vi "TLB Native Dynamic Events ver 0.04e.vi"() -> ()   [LabVIEW 2018]
uses:
  Labview Training Phase 2/Enum Controls/States for Action Engine.ctl
  Type def/TLB event states.ctl
  Type def/TLB MHL States.ctl
  <vilib>/Studica/Studica Toolkit/Background/I2C Channel.ctl
  <vilib>/Studica/Studica Toolkit/NavX/NavX.lvlib
  <vilib>/myRIO/Common/Instrument Driver Framework/myRIO v1.0/AI/typedefs/AI Channels Enum.ctl
  <vilib>/myRIO/Common/Instrument Driver Framework/myRIO v1.0/AI/typedefs/AI Channels List.ctl
  <vilib>/Studica/Studica Toolkit/Background/Mxp Selection.ctl
  <vilib>/ptbypt/NI_PtbyPt.lvlib
panel:
  out "NavX Info Out":T2
  out "LinearAcceleration":T3
  out "Displacement":T4
  out "YRPHfH":T5
  in  "y":dbl=-1.2 format="%#_13g"
  out "Distance":T6
  in  "Return to IDLE":bool
  out "Sharp IR Distance":dbl
  out "Sharp IR Distance 2":dbl
  out "CM":fxp<+,64,16>
  out "Ultrasonic sensor":dbl format="%0.2f"
  out "Waveform Chart 3":dbl(graph)
  in  "xTargetSpeed":dbl
  in  "yTargetSpeed":dbl
  in  "wTargetSpeed":dbl
  out "Speed":T7
  in  "Reset Encoder 0":bool
  out "Action Queue Items":i32
  out "State Logic Queue Items":i32
  out "Action Queues items":string[](array[string])=["Hardware reset", "Software reset", ""]
  out "State logic":T8=enum."Task 2"
  out "Action State":string
  in  "Tasks Selector":string(combo)="Task 2"
  in  "Stop Queue":bool
  in  "Start Task":bool
  # "Test Programme written by Calvin Loke    Dated: 28 Aug 2019\nTest Programme revised by Dr Alex See   Dated 30 Aug 2019\n\nProgramme version:   TLB Native Dynamic Events ver 0.04b.vi"
  # "System Health Status Update"
  # "Sequence of Actions"
  # "Continuous (Repeated)"
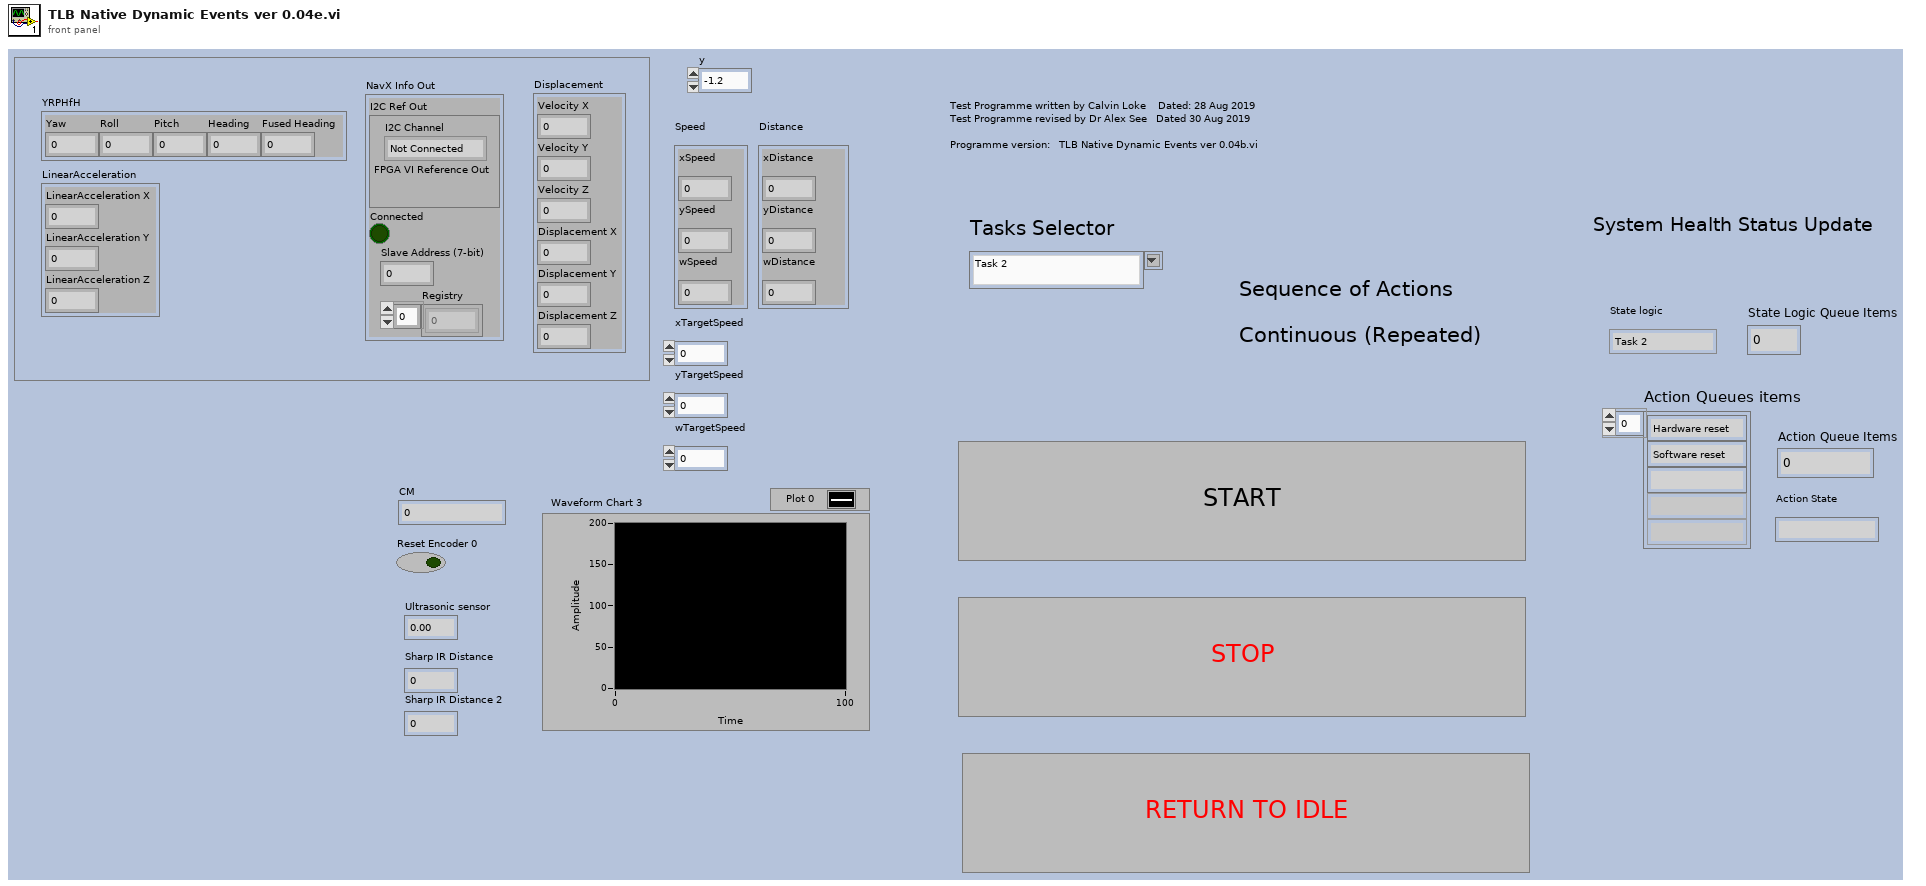
[diagram p1: front panel]
types:
  T1 = typedef "I2C Channel.ctl" = enum16{"Not Connected", "A", "B"}
  T2 = cluster{"I2C Ref Out":cluster{"I2C Channel":T1, "FPGA VI Reference Out":refnum<k20>}, "Connected":bool, "Slave Address (7-bit)":u8, "Registry":u8[]}
  T3 = cluster{"LinearAcceleration X":dbl, "LinearAcceleration Y":dbl, "LinearAcceleration Z":dbl}
  T4 = cluster{"Velocity X":dbl, "Velocity Y":dbl, "Velocity Z":dbl, "Displacement X":dbl, "Displacement Y":dbl, "Displacement Z":dbl}
  T5 = cluster{"Yaw":dbl, "Roll":dbl, "Pitch":dbl, "Heading":dbl, "Fused Heading":dbl}
  T6 = cluster{"xDistance":dbl, "yDistance":dbl, "wDistance":dbl}
  T7 = cluster{"xSpeed":dbl, "ySpeed":dbl, "wSpeed":dbl}
  T8 = typedef "TLB MHL States.ctl" = enum16{"None", "Startup", "Idle", "Processing", "Shutdown", "Reset", "Task 1", "Task 2", "Task 3", "Task 4", "Task 4a", "Task 4b", "Task 4c", "Task 4d", "Task 4e", "Task 4f", "Task 4g", "Task 4h", "Acquire image", "Wall follow mode", "Autodrive", "Autodrive a"}
  T9 = typedef "States for Action Engine.ctl" = enum16{"Initialize", "Write", "Read"}
  T10 = typedef "TLB event states.ctl" = enum16{"Start Sequence", "Exit", "Start Task 1", "Start Task 2", "Start Task 3", "Start Task 4", "Camera vision", "Wall follow mode", "Idle", "Start Drive Straight"}
  T11 = typedef "Mxp Selection.ctl" = enum16{"MXP A", "MXP B"}
  T12 = typedef "TLB event states.ctl" = enum16{"Start Sequence", "Exit", "Task 1", "Task 2", "Task 3", "Idle"}
  T13 = typedef "AI Channels List.ctl" = T14[]
  T14 = typedef "AI Channels Enum.ctl" = enum16{"Not Connected", "AudioIn/Left", "AudioIn/Right", "C/AI0", "C/AI1", "A/AI0", "A/AI1", "A/AI2", "A/AI3", "A/AI4", "A/AI5", "A/AI6", "A/AI7", "B/AI0", "B/AI1", "B/AI2", "B/AI3", "B/AI4", "B/AI5", "B/AI6", "B/AI7", "AI/AI0", "AI/AI1", "AI/AI2", "AI/AI3", "A/AI0 (DIFF)", "A/AI1 (DIFF)", "A/AI2 (DIFF)", "A/AI3 (DIFF)", "B/AI0 (DIFF)", "B/AI1 (DIFF)", "B/AI2 (DIFF)", "B/AI3 (DIFF)"}
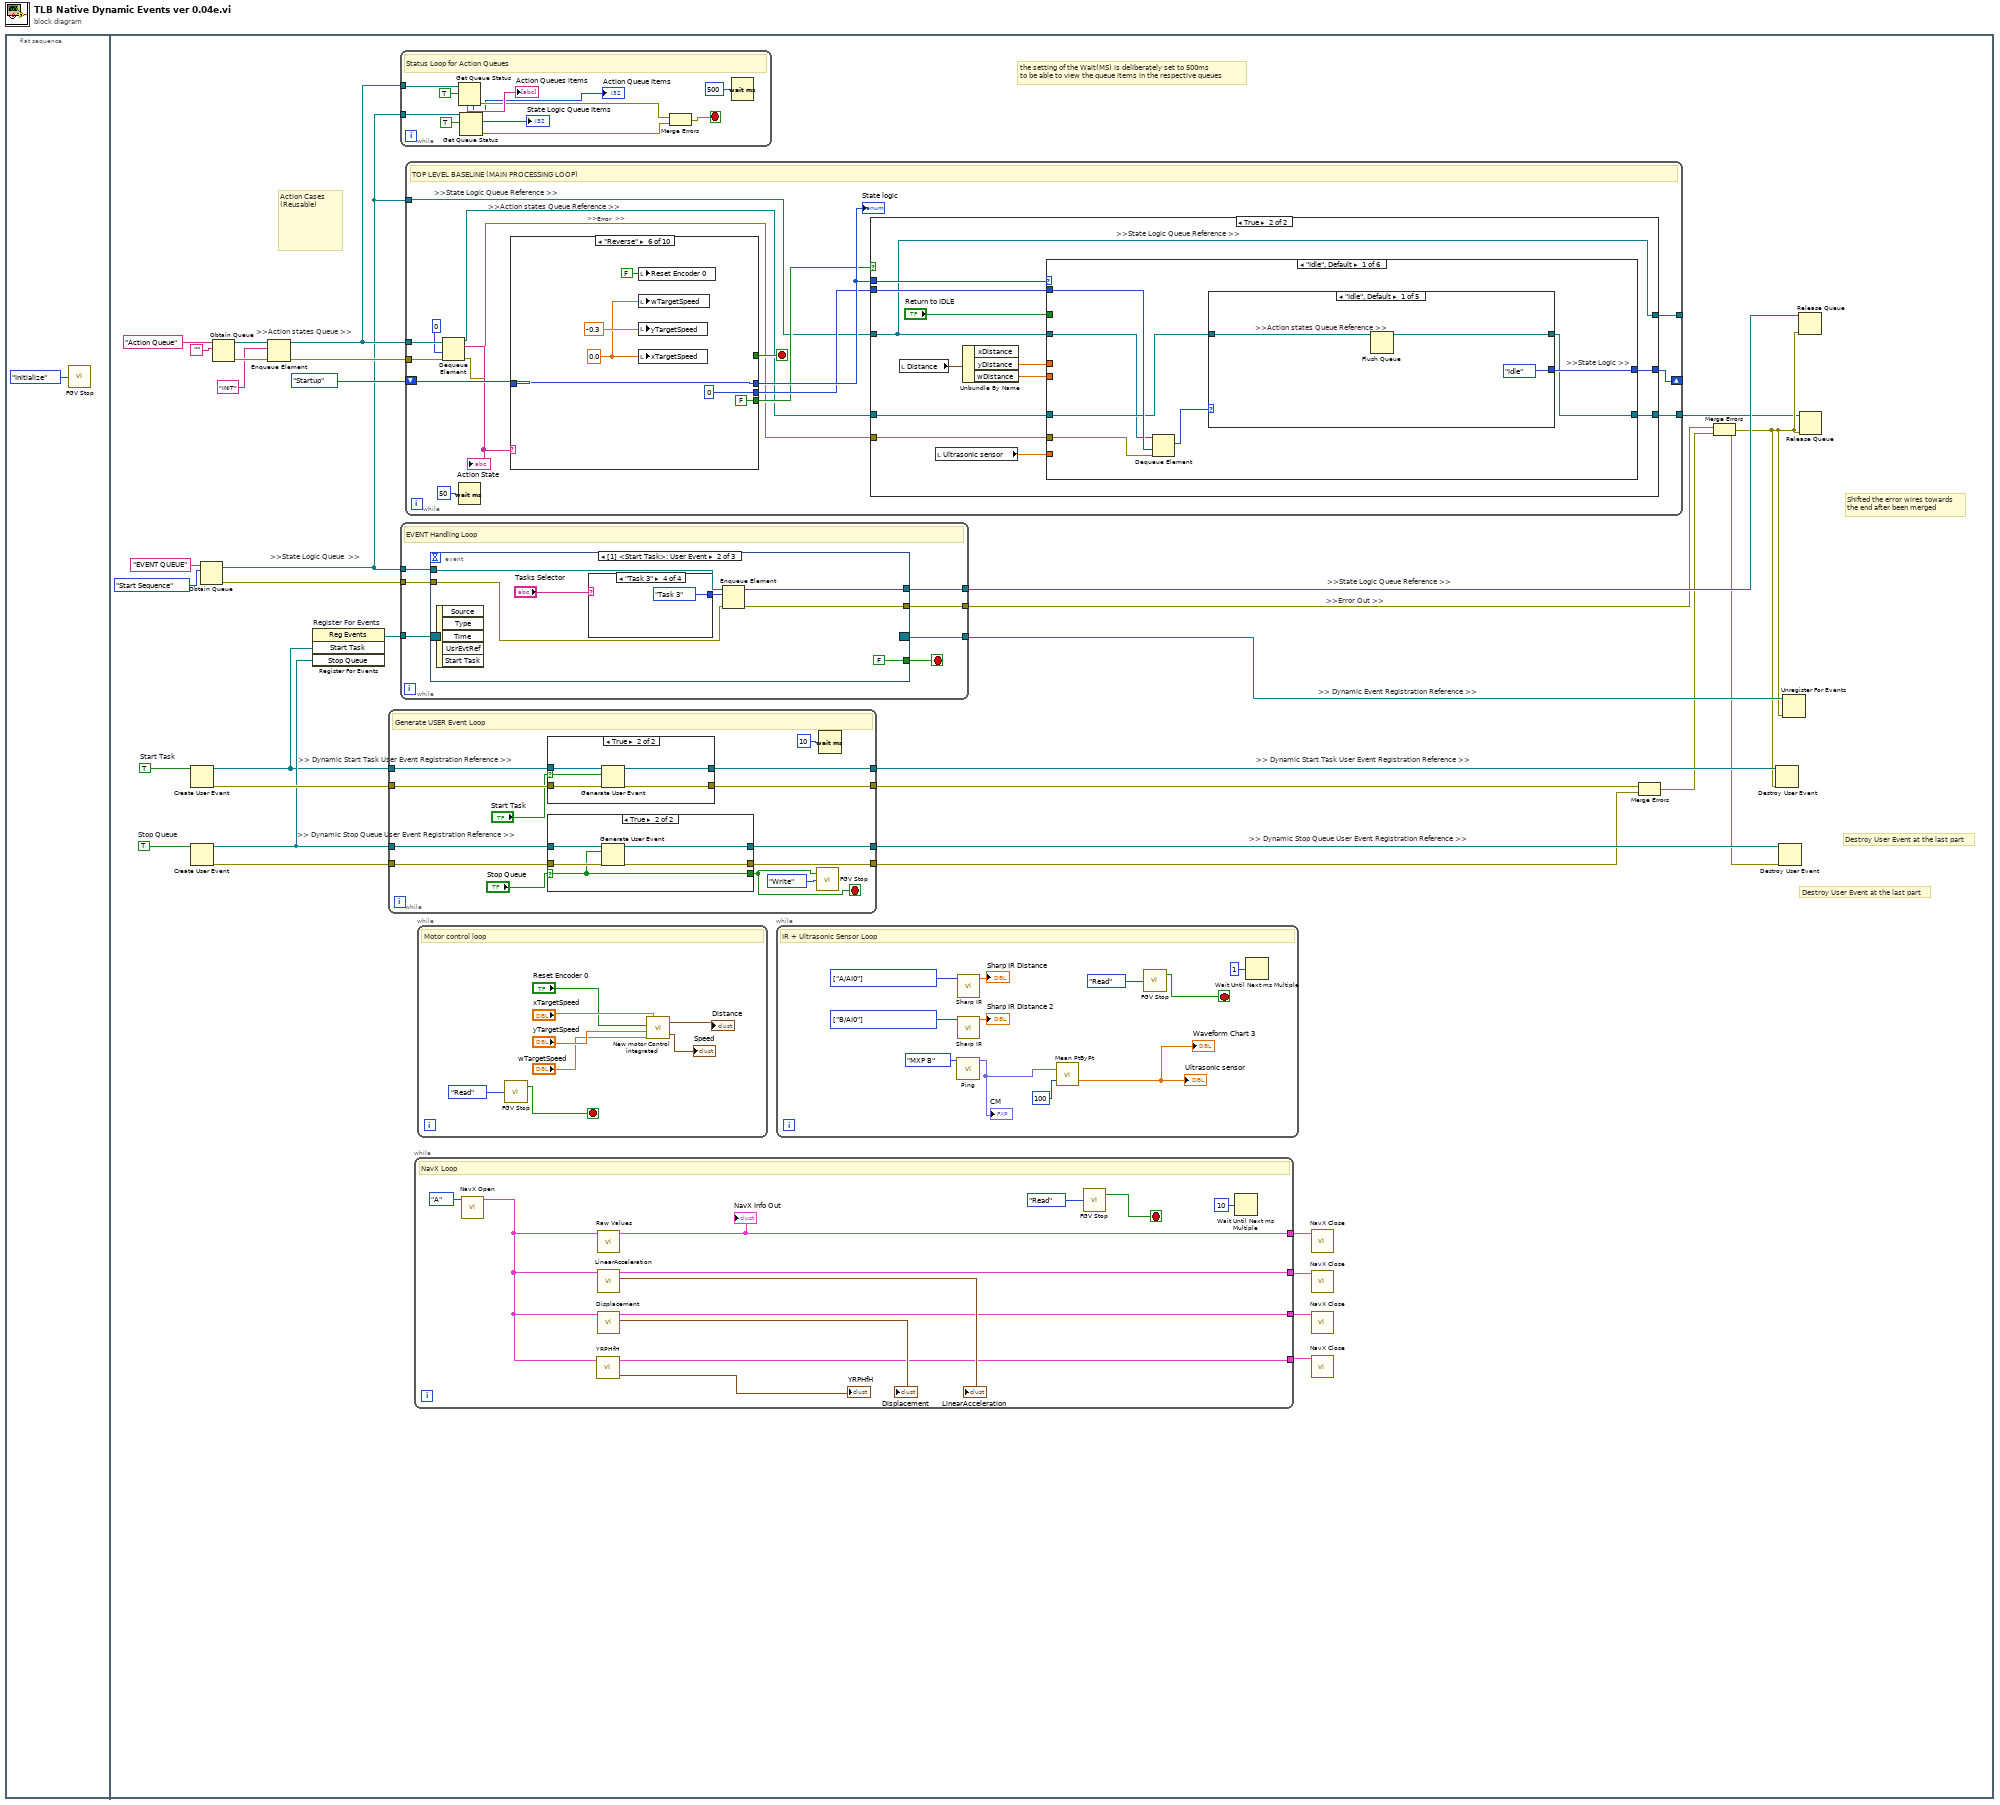
[diagram p0: block diagram]
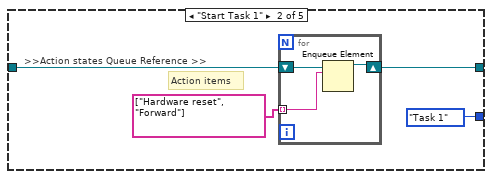
[diagram p3: hidden frame]
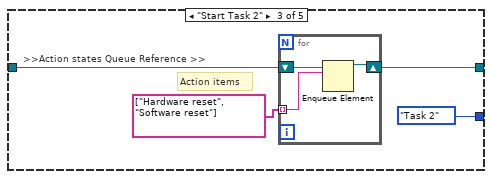
[diagram p4: hidden frame]
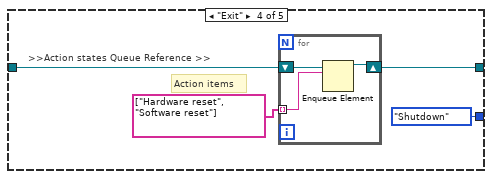
[diagram p5: hidden frame]
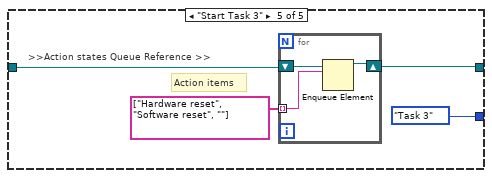
[diagram p6: hidden frame]
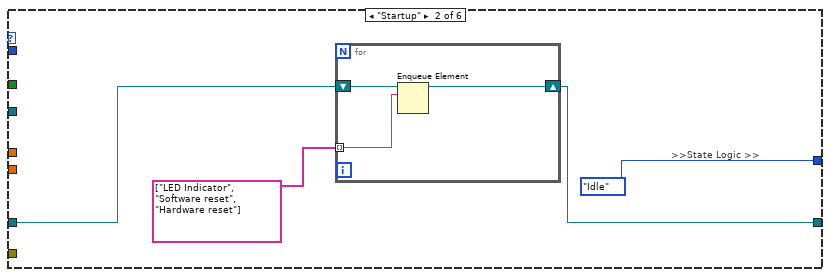
[diagram p7: hidden frame]
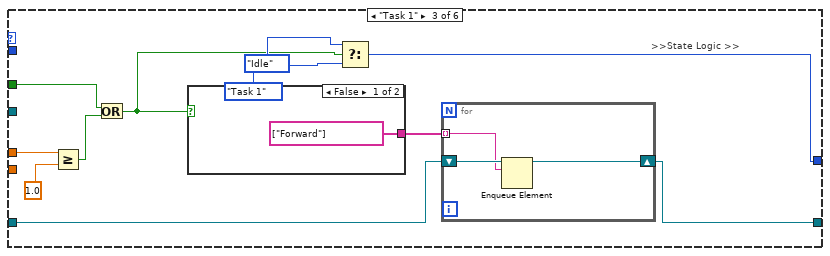
[diagram p8: hidden frame]
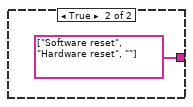
[diagram p9: hidden frame]
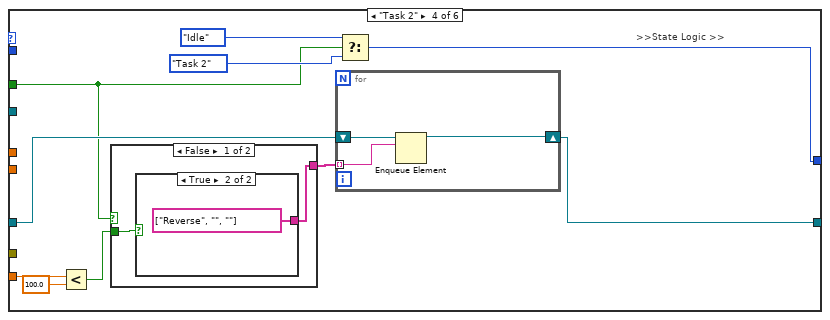
[diagram p10: hidden frame]
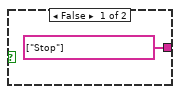
[diagram p11: hidden frame]
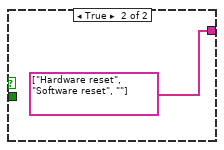
[diagram p12: hidden frame]
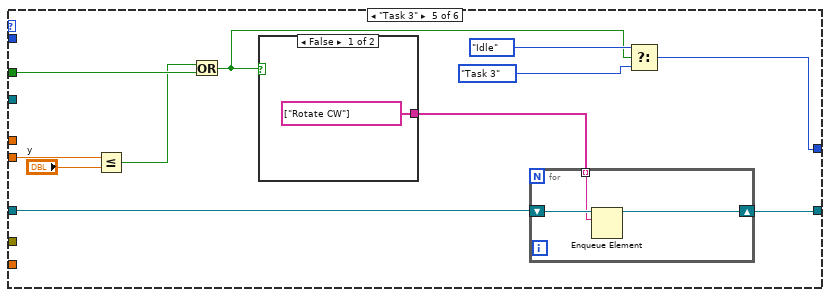
[diagram p13: hidden frame]
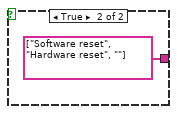
[diagram p14: hidden frame]
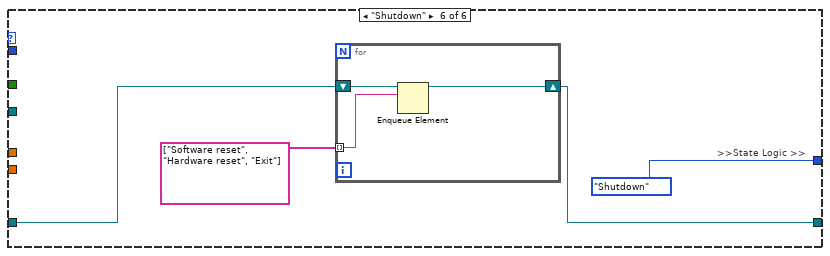
[diagram p15: hidden frame]
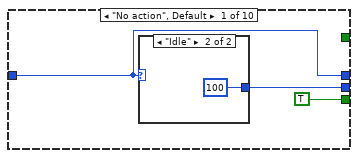
[diagram p16: hidden frame]
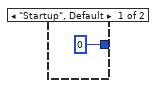
[diagram p17: hidden frame]
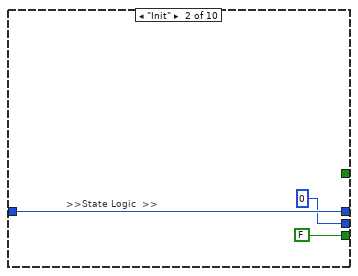
[diagram p18: hidden frame]
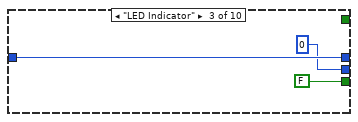
[diagram p19: hidden frame]
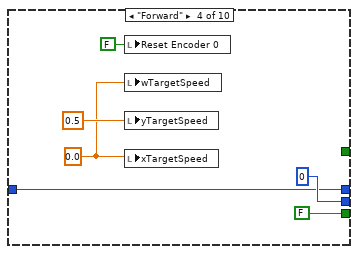
[diagram p20: hidden frame]
diagram:
  n1 = flat-sequence {
    frame #0 {
      n2 = call "FGV Stop.vi"("Init/Read/Write State"=States_for_Action_Engine."Initialize") -> ()  [unwired: 2 in, 2 out]
    }
    frame #1 {
      w34 = TRUE  # Stop Queue
      w33 = TRUE  # Start Task
      # "the setting of the Wait(MS) is deliberately set to 500ms\nto be able to view the queue items in the respective queues"
      # "Action Cases\n(Reusable)"
      # ">>Error Out >>"
      # ">> Dynamic Stop Queue User Event Registration Reference >>"
      # ">> Dynamic Start Task User Event Registration Reference >>"
      # ">> Dynamic Stop Queue User Event Registration Reference >>"
      # ">> Dynamic Start Task User Event Registration Reference >>"
      # ">> Dynamic Event Registration Reference >>"
      # ">>Action states Queue >>"
      # ">>State Logic Queue  >>"
      # ">>State Logic Queue Reference >>"
      # "Destroy User Event at the last part"
      # "Destroy User Event at the last part"
      # "Shifted the error wires towards\nthe end after been merged"
      n3 = Create User Event(user event datatype=w33) -> (user event=w25:refnum<user-event>, error out=w30:errorcluster)  [unwired: 1 in]
      n4 = Create User Event(user event datatype=w34) -> (user event=w26:refnum<user-event>, error out=w29:errorcluster)  [unwired: 1 in]
      n5 = Obtain Queue(name (unnamed)="EVENT QUEUE", element data type=TLB_event_states."Start Sequence" ("Enum")) -> (queue out=w9:refnum<queue>, error out=w15:errorcluster)  [unwired: 3 in, 1 out]
      n6 = Obtain Queue(name (unnamed)="Action Queue", element data type="") -> (queue out=w18:refnum<queue>, error out=w14:errorcluster)  [unwired: 3 in, 1 out]
      n7 = Enqueue Element(queue=w18, element="INIT", error in (no error)=w14) -> (queue out=w10:refnum<queue>, error out=w13:errorcluster)  [unwired: 1 in, 1 out]
      n8 = register-events "Register For Events"(w25, w26) -> (reference out=w24:refnum<event-registration>)  [unwired: 2 in, 1 out]
      n9 = while {
        tunnel: w25 -> [w297]
        tunnel: w26 -> [w296]
        tunnel: [w295] -> w32
        tunnel: [w294] -> w31
        tunnel: w30 -> [w293]
        tunnel: [w292] -> w28
        tunnel: w29 -> [w291]
        tunnel: [w290] -> w27
        stop <- w286 stop-if-true
        # "Generate USER Event Loop"
        n10 = case shown="True" "Start Task" {
          selector: "Start Task" -> [_ w309]
          tunnel: w297 -> [w308 w313]
          tunnel: [w308 w312] -> w294
          tunnel: w293 -> [w307 w311]
          tunnel: [w307 w310] -> w292
          frame False {
          }
          frame True {
            n11 = Generate User Event(user event=w313, event data cluster=w309, error in=w311) -> (user event out=w312:refnum<user-event>, error out=w310:errorcluster)  [unwired: 1 in]
          }
        }
        n12 = case shown="True" "Stop Queue" {
          selector: "Stop Queue" -> [_ w302]
          tunnel: w296 -> [w301 w306]
          tunnel: [w301 w305] -> w295
          tunnel: w291 -> [w300 w304]
          tunnel: [w300 w303] -> w290
          tunnel: [FALSE w302] -> w286
          frame False {
          }
          frame True {
            n13 = Generate User Event(user event=w306, event data cluster=w302, error in=w304) -> (user event out=w305:refnum<user-event>, error out=w303:errorcluster)  [unwired: 1 in]
          }
        }
        n14 = call "FGV Stop.vi"("Init/Read/Write State"=States_for_Action_Engine."Write", "Input Node"=w286) -> ()  [unwired: 1 in, 2 out]
        n15 = Wait (ms)(milliseconds to wait=u32 10) -> ()  [unwired: 1 out]
      }
      n16 = while {
        tunnel: w10 -> [w74]
        tunnel: w9 -> [w71]
        stop <- w68 stop-if-true
        # "Status Loop for Action Queues"
        n17 = Get Queue Status(queue=w74, return elements? (F)=TRUE) -> (error out=w70:errorcluster, # elements in queue=→"Action Queue Items":i32, elements=→"Action Queues items":string[])  [unwired: 1 in, 5 out]
        n18 = Get Queue Status(queue=w71, return elements? (F)=TRUE) -> (# pending remove=→"State Logic Queue Items":i32, error out=w69:errorcluster)  [unwired: 1 in, 6 out]
        n19 = Merge Errors(w70, w69) -> (w68:errorcluster)
        n20 = Wait (ms)(milliseconds to wait=u32 500) -> ()  [unwired: 1 out]
      }
      n21 = while {
        tunnel: w24 -> [w262]
        tunnel: [w261] -> w23
        tunnel: w9 -> [w259]
        tunnel: [w258] -> w22
        tunnel: w15 -> [w257]
        tunnel: [w256] -> w12
        stop <- w260 stop-if-true
        # "EVENT Handling Loop"
        n22 = event shown="[1] <Start Task>: User Event" {
          selector: w262 -> [_ _ _]
          dyn-events: [_ _ _] -> w261
          timeout: _ -> [_ _ _]
          tunnel: [FALSE FALSE w285] -> w260
          tunnel: w259 -> [w267 w274 w283]
          tunnel: [w266 w273 w284] -> w258
          tunnel: w257 -> [w264 w270 w281]
          tunnel: [w263 w269 w280] -> w256
          event Timeout {
            n23 = event-data() -> ()  [unwired: 1 in, 3 out]
            n24 = Enqueue Element(queue=w267, element=TLB_event_states."Idle" ("Enum"), error in (no error)=w264) -> (queue out=w266:refnum<queue>, error out=w263:errorcluster)  [unwired: 1 in, 1 out]
          }
          event User Event {
            n25 = event-data() -> ()  [unwired: 1 in, 5 out]
            n26 = case shown="\"Task 3\"" "Tasks Selector" {
              tunnel: [TLB_event_states."Idle" ("Enum") TLB_event_states."Start Task 1" ("Enum") TLB_event_states."Task 2" ("Enum") TLB_event_states."Task 3" ("Enum")] -> w271
              frame Default {
              }
              frame "Task 1" {
              }
              frame "Task 2" {
              }
              frame "Task 3" {
              }
            }
            n27 = Enqueue Element(queue=w274, element=w271, error in (no error)=w270) -> (queue out=w273:refnum<queue>, error out=w269:errorcluster)  [unwired: 1 in, 1 out]
          }
          event User Event {
            n28 = event-data() -> ("Stop Queue"=w285:bool)  [unwired: 1 in, 4 out]
            n29 = Enqueue Element At Opposite End(queue=w283, element=TLB_event_states."Exit" ("Enum"), error in (no error)=w281) -> (queue out=w284:refnum<queue>, error out=w280:errorcluster)  [unwired: 1 in, 1 out]
          }
        }
      }
      n30 = while {
        tunnel: w9 -> [w79]
        shift-right: [w84] -> _
        shift-left: TLB_MHL_States."Startup" ("Enum") -> [w91]
        tunnel: w10 -> [w89]
        tunnel: w13 -> [w87]
        tunnel: [w86] -> _
        tunnel: [w85] -> w7
        stop <- w82 stop-if-true
        # ">>Error  >>"
        # ">>Action states Queue Reference >>"
        # ">>State Logic Queue Reference >>"
        # "TOP LEVEL BASELINE (MAIN PROCESSING LOOP)"
        n31 = Dequeue Element(queue=w89, timeout in ms (-1)=0, error in (no error)=w87) -> (queue out=w78:refnum<queue>, element=w88:string, error out=w77:errorcluster)  [unwired: 1 out]
        "Action State" <- w88
        n32 = Wait (ms)(milliseconds to wait=u32 50) -> ()  [unwired: 1 out]
        n33 = case shown="\"Reverse\"" w88 {
          tunnel: [w212 w217 w220 w225 w230 w237 w242 w246 w251 TLB_MHL_States."Shutdown" ("Enum")] -> w90
          tunnel: w91 -> [w212 w217 w220 w225 w230 w237 w242 w246 w251 _]
          tunnel: [w211 0 0 0 0 0 0 0 0 0] -> w83
          tunnel: [_ _ _ _ _ _ _ _ _ TRUE] -> w82
          tunnel: [TRUE FALSE FALSE FALSE FALSE FALSE FALSE FALSE FALSE FALSE] -> w81
          frame "No action", Default {
            n34 = case shown="\"Idle\"" w212 {
              tunnel: [0 100] -> w211
              frame "Startup", Default {
              }
              frame "Idle" {
              }
            }
          }
          frame "Init" {
            # ">>State Logic  >>"
          }
          frame "LED Indicator" {
          }
          frame "Forward" {
            w221 = 0.0
            n35 = local write "Reset Encoder 0"(FALSE ("Reset Encoder 0")) -> ()
            n36 = local write "wTargetSpeed"(w221) -> ()
            n37 = local write "yTargetSpeed"(0.5 ("yTargetSpeed")) -> ()
            n38 = local write "xTargetSpeed"(w221) -> ()
          }
          frame "Rotate CW" {
            w227 = 0.0
            n39 = local write "Reset Encoder 0"(FALSE ("Reset Encoder 0")) -> ()
            n40 = local write "wTargetSpeed"(-0.15 ("yTargetSpeed")) -> ()
            n41 = local write "yTargetSpeed"(w227) -> ()
            n42 = local write "xTargetSpeed"(w227) -> ()
          }
          frame "Reverse" {
            w233 = 0.0
            n43 = local write "Reset Encoder 0"(FALSE ("Reset Encoder 0")) -> ()
            n44 = local write "wTargetSpeed"(w233) -> ()
            n45 = local write "yTargetSpeed"(-0.3 ("yTargetSpeed")) -> ()
            n46 = local write "xTargetSpeed"(w233) -> ()
          }
          frame "Stop" {
            w239 = 0.0
            n47 = local write "Reset Encoder 0"(FALSE ("Reset Encoder 0")) -> ()
            n48 = local write "wTargetSpeed"(w239) -> ()
            n49 = local write "yTargetSpeed"(w239) -> ()
            n50 = local write "xTargetSpeed"(w239) -> ()
          }
          frame "Software reset" {
          }
          frame "Hardware reset" {
            w247 = 0.0
            n51 = local write "Reset Encoder 0"(TRUE ("Reset Encoder 0")) -> ()
            n52 = local write "wTargetSpeed"(w247) -> ()
            n53 = local write "yTargetSpeed"(w247) -> ()
            n54 = local write "xTargetSpeed"(w247) -> ()
          }
          frame "Exit" {
          }
        }
        "State logic" <- w90
        n55 = case shown="True" w81 {
          tunnel: w90 -> [w94 w107]
          tunnel: w79 -> [w95 w101]
          tunnel: w78 -> [w93 w106]
          tunnel: [w95 w101] -> w86
          tunnel: [w93 w105] -> w85
          tunnel: [w94 w104] -> w84
          tunnel: w77 -> [_ w103]
          tunnel: w83 -> [_ w102]
          frame False {
          }
          frame True {
            # ">>State Logic Queue Reference >>"
            n56 = local read "Distance"() -> (w99:T6)
            n57 = local read "Ultrasonic sensor"() -> (w97:dbl)
            n58 = Unbundle By Name(w99) -> ("yDistance"=w98:dbl, "wDistance"=w96:dbl)  [unwired: 1 out]
            n59 = case shown="\"Idle\", Default" w107 {
              tunnel: w101 -> [w108 _ _ _ _ _]
              tunnel: w106 -> [w110 w147 w159 w174 w196 w204]
              tunnel: [w109 w146 w158 w175 w195 w203] -> w105
              tunnel: [w113 TLB_MHL_States."Idle" ("Enum") w161 w176 w192 TLB_MHL_States."Shutdown" ("Enum")] -> w104
              tunnel: w103 -> [w111 _ _ _ _ _]
              tunnel: w102 -> [w112 _ _ _ _ _]
              tunnel: "Return to IDLE" -> [_ _ w156 w171 w190 _]
              tunnel: w98 -> [_ _ w155 _ _ _]
              tunnel: w97 -> [_ _ _ w173 _ _]
              tunnel: w96 -> [_ _ _ _ w189 _]
              frame "Idle", Default {
                # ">>State Logic >>"
                n60 = Dequeue Element(queue=w108, timeout in ms (-1)=w112, error in (no error)=w111) -> (element=w114:T10)  [unwired: 3 out]
                n61 = case shown="\"Idle\", Default" w114 {
                  tunnel: [TLB_MHL_States."Idle" ("Enum") TLB_MHL_States."Task 1" ("Enum") TLB_MHL_States."Task 2" ("Enum") TLB_MHL_States."Shutdown" ("Enum") TLB_MHL_States."Task 3" ("Enum")] -> w113
                  tunnel: [w115 w120 w125 w132 w141] -> w109
                  tunnel: w110 -> [w116 w118 w126 w133 w142]
                  frame "Idle", Default {
                    # ">>Action states Queue Reference >>"
                    n62 = Flush Queue(queue=w116) -> (queue out=w115:refnum<queue>)  [unwired: 1 in, 2 out]
                  }
                  frame "Start Task 1" {
                    # ">>Action states Queue Reference >>"
                    # "Action items"
                    n63 = for {
                      shift-right: [w124] -> w120
                      shift-left: w118 -> [w123]
                      tunnel: string[] ["Hardware reset", "Forward"] -> [w122] mode=indexing
                      n64 = Enqueue Element(queue=w123, element=w122) -> (queue out=w124:refnum<queue>)  [unwired: 2 in, 2 out]
                    }
                  }
                  frame "Start Task 2" {
                    # ">>Action states Queue Reference >>"
                    # "Action items"
                    n65 = for {
                      shift-right: [w131] -> w125
                      shift-left: w126 -> [w130]
                      tunnel: string[] ["Hardware reset", "Software reset"] -> [w129] mode=indexing
                      n66 = Enqueue Element(queue=w130, element=w129) -> (queue out=w131:refnum<queue>)  [unwired: 2 in, 2 out]
                    }
                  }
                  frame "Exit" {
                    # ">>Action states Queue Reference >>"
                    # "Action items"
                    n67 = for {
                      shift-right: [w138] -> w132
                      shift-left: w133 -> [w137]
                      tunnel: string[] ["Hardware reset", "Software reset"] -> [w136] mode=indexing
                      n68 = Enqueue Element(queue=w137, element=w136) -> (queue out=w138:refnum<queue>)  [unwired: 2 in, 2 out]
                    }
                  }
                  frame "Start Task 3" {
                    # ">>Action states Queue Reference >>"
                    # "Action items"
                    n69 = for {
                      shift-right: [w145] -> w141
                      shift-left: w142 -> [w144]
                      tunnel: string[] ["Hardware reset", "Software reset", ""] -> [w143] mode=indexing
                      n70 = Enqueue Element(queue=w144, element=w143) -> (queue out=w145:refnum<queue>)  [unwired: 2 in, 2 out]
                    }
                  }
                }
              }
              frame "Startup" {
                # ">>State Logic >>"
                n71 = for {
                  shift-right: [w151] -> w146
                  shift-left: w147 -> [w152]
                  tunnel: string[] ["LED Indicator", "Software reset", "Hardware reset"] -> [w150] mode=indexing
                  n72 = Enqueue Element(queue=w152, element=w150) -> (queue out=w151:refnum<queue>)  [unwired: 2 in, 2 out]
                }
              }
              frame "Task 1" {
                # ">>State Logic >>"
                n73 = Greater Or Equal?(x=w155, y=1.0) -> (x >= y?=w153:bool)
                n74 = Or(x=w156, y=w153) -> (x .or. y?=w157:bool)
                n75 = case shown="False" w157 {
                  tunnel: [string[] ["Forward"] string[] ["Software reset", "Hardware reset", ""]] -> w160
                  frame False {
                  }
                  frame True {
                  }
                }
                n76 = Select(t=TLB_MHL_States."Idle" ("Enum"), s=w157, f=TLB_MHL_States."Task 1" ("Enum")) -> (s? t:f=w161:T8)
                n77 = for {
                  shift-right: [w167] -> w158
                  shift-left: w159 -> [w168]
                  tunnel: w160 -> [w166] mode=indexing
                  n78 = Enqueue Element(queue=w168, element=w166) -> (queue out=w167:refnum<queue>)  [unwired: 2 in, 2 out]
                }
              }
              frame "Task 2" {
                # ">>State Logic >>"
                n79 = Less?(x=w173, y=100.0) -> (x < y?=w169:bool)
                n80 = case shown="False" w171 {
                  tunnel: [w179 string[] ["Hardware reset", "Software reset", ""]] -> w170
                  tunnel: w169 -> [w180 _]
                  frame False {
                    n81 = case shown="True" w180 {
                      tunnel: [string[] ["Stop"] string[] ["Reverse", "", ""]] -> w179
                      frame False {
                      }
                      frame True {
                      }
                    }
                  }
                  frame True {
                  }
                }
                n82 = for {
                  shift-right: [w185] -> w175
                  shift-left: w174 -> [w186]
                  tunnel: w170 -> [w184] mode=indexing
                  n83 = Enqueue Element(queue=w186, element=w184) -> (queue out=w185:refnum<queue>)  [unwired: 2 in, 2 out]
                }
                n84 = Select(t=TLB_MHL_States."Idle" ("Enum"), s=w171, f=TLB_MHL_States."Task 2" ("Enum")) -> (s? t:f=w176:T8)
              }
              frame "Task 3" {
                n85 = Less Or Equal?(x=w189, y="y") -> (x <= y?=w187:bool)
                n86 = Or(x=w187, y=w190) -> (x .or. y?=w191:bool)
                n87 = case shown="False" w191 {
                  tunnel: [string[] ["Rotate CW"] string[] ["Software reset", "Hardware reset", ""]] -> w197
                  frame False {
                  }
                  frame True {
                  }
                }
                n88 = for {
                  shift-right: [w199] -> w195
                  shift-left: w196 -> [w200]
                  tunnel: w197 -> [w198] mode=indexing
                  n89 = Enqueue Element(queue=w200, element=w198) -> (queue out=w199:refnum<queue>)  [unwired: 2 in, 2 out]
                }
                n90 = Select(t=TLB_MHL_States."Idle" ("Enum"), s=w191, f=TLB_MHL_States."Task 3" ("Enum")) -> (s? t:f=w192:T8)
              }
              frame "Shutdown" {
                # ">>State Logic >>"
                n91 = for {
                  shift-right: [w208] -> w203
                  shift-left: w204 -> [w209]
                  tunnel: string[] ["Software reset", "Hardware reset", "Exit"] -> [w207] mode=indexing
                  n92 = Enqueue Element(queue=w209, element=w207) -> (queue out=w208:refnum<queue>)  [unwired: 2 in, 2 out]
                }
              }
            }
          }
        }
      }
      n93 = while {
        tunnel: [w54] -> w5
        tunnel: [w50] -> w4
        tunnel: [w49] -> w2
        tunnel: [w48] -> w3
        stop <- w56 stop-if-true
        # "NavX Loop"
        n94 = call <vilib>:"NavX Open.vi"("I2C Channel"=I2C_Channel."A") -> ("NavX Info"=w46:T2)  [unwired: 9 in, 1 out]
        n95 = call <vilib>:"YRPHfH.vi"("NavX Info In"=w46) -> ("YRPHfH"=→"YRPHfH":T5, "NavX Info Out"=w49:T2)  [unwired: 3 in]
        n96 = call <vilib>:"Raw Values.vi"("NavX Info In"=w46) -> ("NavX Info Out"=w54:T2)  [unwired: 8 in, 1 out]
        "NavX Info Out" <- w54
        n97 = call <vilib>:"LinearAcceleration.vi"("NavX Info In"=w46) -> ("LinearAcceleration"=→"LinearAcceleration":T3, "NavX Info Out"=w50:T2)  [unwired: 9 in]
        n98 = call <vilib>:"Displacement.vi"("NavX Info In"=w46) -> ("Displacement"=→"Displacement":T4, "NavX Info Out"=w48:T2)  [unwired: 9 in]
        n99 = call "FGV Stop.vi"("Init/Read/Write State"=States_for_Action_Engine."Read") -> ("Output node"=w56:bool)  [unwired: 2 in, 1 out]
        n100 = Wait Until Next ms Multiple(millisecond multiple=u32 10) -> ()  [unwired: 1 out]
      }
      n101 = while {
        stop <- w64 stop-if-true
        # "Motor control loop"
        n102 = call "FGV Stop.vi"("Init/Read/Write State"=States_for_Action_Engine."Read") -> ("Output node"=w64:bool)  [unwired: 2 in, 1 out]
        n103 = call "New motor Control integrated.vi"("wTargetSpeed"="wTargetSpeed", "yTargetSpeed"="yTargetSpeed", "xTargetSpeed"="Reset Encoder 0", "Reset Encoders"="xTargetSpeed") -> ("Speed"=→"Speed":T7, "Distance"=→"Distance":T6)
      }
      n104 = while {
        stop <- w39 stop-if-true
        w44 = T13 [enum."B/AI0"] items=["Not Connected", "AudioIn/Left", "AudioIn/Right", "C/AI0", "C/AI1", "A/AI0", "A/AI1", "A/AI2", "A/AI3", "A/AI4", "A/AI5", "A/AI6", "A/AI7", "B/AI0", "B/AI1", "B/AI2", "B/AI3", "B/AI4", "B/AI5", "B/AI6", "B/AI7", "AI/AI0", "AI/AI1", "AI/AI2", "AI/AI3", "A/AI0 (DIFF)", "A/AI1 (DIFF)", "A/AI2 (DIFF)", "A/AI3 (DIFF)", "B/AI0 (DIFF)", "B/AI1 (DIFF)", "B/AI2 (DIFF)", "B/AI3 (DIFF)"] ("AI Channel")
        w45 = T13 [enum."A/AI0"] items=["Not Connected", "AudioIn/Left", "AudioIn/Right", "C/AI0", "C/AI1", "A/AI0", "A/AI1", "A/AI2", "A/AI3", "A/AI4", "A/AI5", "A/AI6", "A/AI7", "B/AI0", "B/AI1", "B/AI2", "B/AI3", "B/AI4", "B/AI5", "B/AI6", "B/AI7", "AI/AI0", "AI/AI1", "AI/AI2", "AI/AI3", "A/AI0 (DIFF)", "A/AI1 (DIFF)", "A/AI2 (DIFF)", "A/AI3 (DIFF)", "B/AI0 (DIFF)", "B/AI1 (DIFF)", "B/AI2 (DIFF)", "B/AI3 (DIFF)"] ("AI Channel")
        # "IR + Ultrasonic Sensor Loop"
        n105 = call <vilib>:"Ping.vi"("Mxp Side"=Mxp_Selection."MXP B") -> ("CM"=w35:fxp<+,64,16>)  [unwired: 8 in, 2 out]
        "CM" <- w35
        n106 = call <vilib>:"Sharp IR.vi"("AI Channel"=w45) -> ("Sharp IR Distance"=→"Sharp IR Distance":dbl)  [unwired: 8 in, 2 out]
        n107 = call <vilib>:"Sharp IR.vi"("AI Channel"=w44) -> ("Sharp IR Distance"=→"Sharp IR Distance 2":dbl)  [unwired: 8 in, 2 out]
        n108 = call <vilib>:"Mean PtByPt.vi"("x"=w35, "sample length"=100) -> ("mean"=→"Ultrasonic sensor" →"Waveform Chart 3":dbl)  [unwired: 2 in, 1 out]
        n109 = call "FGV Stop.vi"("Init/Read/Write State"=States_for_Action_Engine."Read") -> ("Output node"=w39:bool)  [unwired: 2 in, 1 out]
        n110 = Wait Until Next ms Multiple(millisecond multiple=u32 1) -> ()  [unwired: 1 out]
      }
      n111 = call <vilib>:"NavX Close.vi"("NavX Info In"=w5) -> ()  [unwired: 10 in, 1 out]
      n112 = call <vilib>:"NavX Close.vi"("NavX Info In"=w4) -> ()  [unwired: 10 in, 1 out]
      n113 = call <vilib>:"NavX Close.vi"("NavX Info In"=w3) -> ()  [unwired: 10 in, 1 out]
      n114 = call <vilib>:"NavX Close.vi"("NavX Info In"=w2) -> ()  [unwired: 10 in, 1 out]
      n115 = Merge Errors "Merge Errors"(w28, w27) -> (w6:errorcluster)
      n116 = Merge Errors(w12, w6) -> (w8:errorcluster)
      n117 = Destroy User Event(user event=w31, error in=w8) -> ()  [unwired: 1 out]
      n118 = Destroy User Event(user event=w32, error in=w8) -> ()  [unwired: 1 out]
      n119 = Unregister For Events(event registration refnum=w23, error in=w8) -> ()  [unwired: 1 out]
      n120 = Release Queue(queue=w22, error in (no error)=w8) -> ()  [unwired: 1 in, 3 out]
      n121 = Release Queue(queue=w7, error in (no error)=w8) -> ()  [unwired: 1 in, 3 out]
    }
  }
